vi "Handle Value Change.vi"(5 "VolatusAPI":refnum<class "VolatusAPI.lvclass">, 7 "CtlRef":refnum<vi>, 8 "error in (no error)":errorcluster, 9 "NewVal":variant, 10 "OldVal":variant, 11 "Sequencing Control in":refnum<class "Sequencing Control.lvclass">) -> (0 "error out":errorcluster, 3 "Sequencing Control out":refnum<class "Sequencing Control.lvclass">)   [LabVIEW 2020, in "VolatusSeqGUI.lvlib" / "Sequencing Control.lvclass"]
uses:
  Sequencing Control.lvclass
  Volatus/VolatusAPI/VolatusAPI.lvclass
  Action.ctl
  Action Data.ctl
  Sequencing Control.lvclass/Sequencing Control.ctl
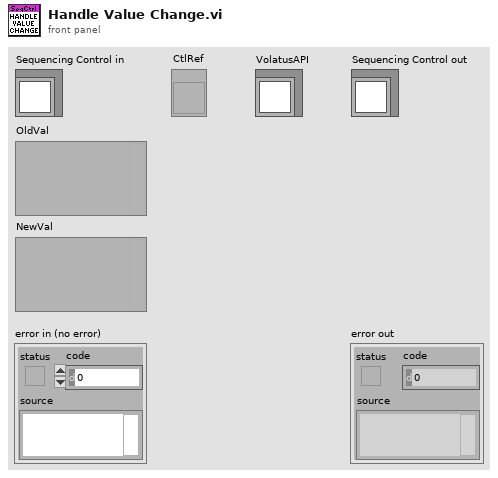
[diagram p1: front panel]
types:
  T1 = cluster{"Sequences":cluster{"Name Color":u32, "Name":string, "Btn 1 Color":u32, "Btn 1 Text":string, "Btn 2 Color":u32, "Btn 2 Text":string, "Status Color":u32, "Status":string, "State Time":string, "Started":string, "Seq Time":string, "Btn 1":bool, "Btn 2":bool, "Btn Name":bool}[], "Unload All":bool, "Abort All":bool, "Loaded, Good CRC":u32, "Sequence Error":u32, "Loaded, CRC Mismatch":u32, "Running, Good CRC":u32, "Unloaded":u32, "Running, CRC Mismatch":u32}
  T2 = cluster{"Sequences":cluster{"Name Color":bool, "Name":bool, "Btn 1 Color":bool, "Btn 1 Text":bool, "Btn 2 Color":bool, "Btn 2 Text":bool, "Status Color":bool, "Status":bool, "State Time":bool, "Started":bool, "Seq Time":bool, "Btn 1":bool, "Btn 2":bool, "Btn Name":bool}[], "Unload All":bool, "Abort All":bool, "Loaded, Good CRC":bool, "Sequence Error":bool, "Loaded, CRC Mismatch":bool, "Running, Good CRC":bool, "Unloaded":bool, "Running, CRC Mismatch":bool}
  T3 = cluster{"Name Color":u32, "Name":string, "Btn 1 Color":u32, "Btn 1 Text":string, "Btn 2 Color":u32, "Btn 2 Text":string, "Status Color":u32, "Status":string, "State Time":string, "Started":string, "Seq Time":string, "Btn 1":bool, "Btn 2":bool, "Btn Name":bool}[]
  T4 = cluster{"Name Color":bool, "Name":bool, "Btn 1 Color":bool, "Btn 1 Text":bool, "Btn 2 Color":bool, "Btn 2 Text":bool, "Status Color":bool, "Status":bool, "State Time":bool, "Started":bool, "Seq Time":bool, "Btn 1":bool, "Btn 2":bool, "Btn Name":bool}[]
  T5 = typedef "VolatusSeqGUI.lvlib/Sequencing Control.lvclass/Action.ctl" = enum16{"Details", "Load", "Unload", "Run", "Abort", "Unload All", "Abort All"}
  T6 = typedef "VolatusSeqGUI.lvlib/Sequencing Control.lvclass/Action Data.ctl" = cluster{"Action":T5, "Sequence":string}
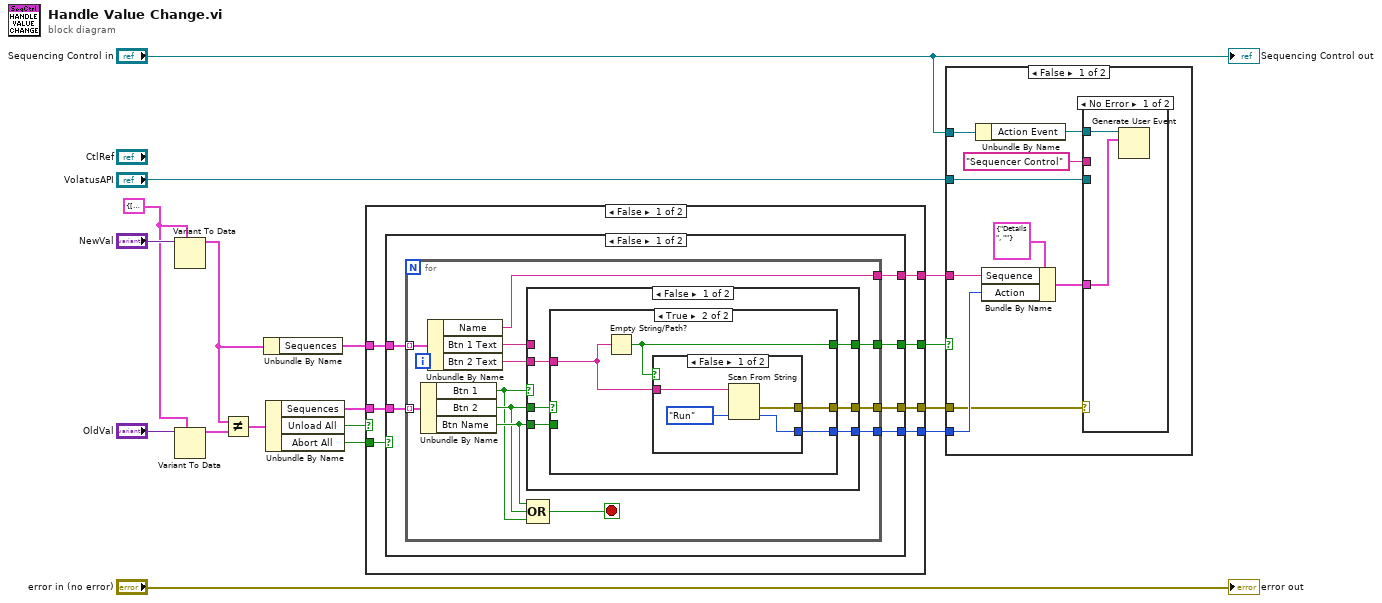
[diagram p0: block diagram]
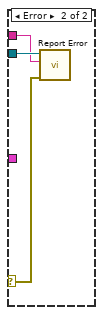
[diagram p2: hidden frame]
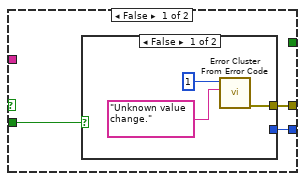
[diagram p4: hidden frame]
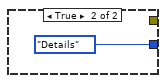
[diagram p5: hidden frame]
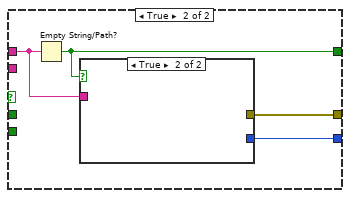
[diagram p7: hidden frame]
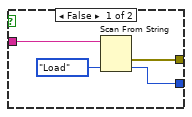
[diagram p8: hidden frame]
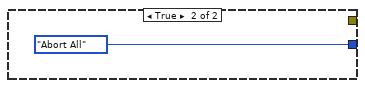
[diagram p9: hidden frame]
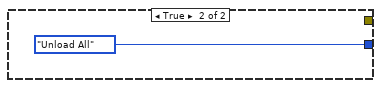
[diagram p10: hidden frame]
diagram:
  w14 = T1 {"Sequences"=[], "Unload All"=FALSE, "Abort All"=FALSE, "Loaded, Good CRC"=13816530, "Sequence Error"=16744319, "Loaded, CRC Mismatch"=16777142, "Running, Good CRC"=11730866, "Unloaded"=7171459, "Running, CRC Mismatch"=10530559} ("Sequencing")
  n1 = Variant To Data(type=w14, Variant="NewVal") -> (data=w8:T1)  [unwired: 1 in, 1 out]
  n2 = Variant To Data(type=w14, Variant="OldVal") -> (data=w13:T1)  [unwired: 1 in, 1 out]
  n3 = Not Equal?(x=w8, y=w13) -> (x != y?=w12:T2)
  n4 = Unbundle By Name(w8) -> ("Sequences"=w7:T3)
  n5 = Unbundle By Name(w12) -> ("Sequences"=w9:T4, "Unload All"=w11:bool, "Abort All"=w10:bool)
  n6 = case shown="False" w11 {
    tunnel: w10 -> [w24 _]
    tunnel: w9 -> [w22 _]
    tunnel: [w23 Action."Unload All" ("Action")] -> w5
    tunnel: w7 -> [w21 _]
    tunnel: [w20 _] -> w6
    tunnel: [w19 _] -> w3
    tunnel: [w18 _] -> w1
    frame False {
      n7 = case shown="False" w24 {
        tunnel: [w27 Action."Abort All" ("Action")] -> w23
        tunnel: w22 -> [w30 _]
        tunnel: w21 -> [w29 _]
        tunnel: [w28 _] -> w20
        tunnel: [w26 _] -> w19
        tunnel: [w25 _] -> w18
        frame False {
          n8 = for {
            tunnel: w30 -> [w42] mode=indexing
            tunnel: w29 -> [w41] mode=indexing
            tunnel: [w38] -> w28
            tunnel: [w37] -> w27
            tunnel: [w36] -> w26
            tunnel: [w31] -> w25
            stop <- w32 stop-if-true
            n9 = Unbundle By Name(w42) -> ("Btn 1"=w33:bool, "Btn 2"=w34:bool, "Btn Name"=w35:bool)
            n10 = Unbundle By Name(w41) -> ("Name"=w38:string, "Btn 1 Text"=w40:string, "Btn 2 Text"=w39:string)
            n11 = case shown="False" w33 {
              tunnel: w39 -> [w47 _]
              tunnel: [w44 w67] -> w37
              tunnel: [w46 w66] -> w36
              tunnel: w40 -> [_ w65]
              tunnel: w34 -> [w48 _]
              tunnel: w35 -> [w45 _]
              tunnel: [w43 w64] -> w31
              frame False {
                n12 = case shown="True" w48 {
                  tunnel: w47 -> [_ w57]
                  tunnel: [w49 w59] -> w46
                  tunnel: w45 -> [w51 _]
                  tunnel: [w50 w58] -> w44
                  tunnel: [_ w56] -> w43
                  frame False {
                    n13 = case shown="False" w51 {
                      tunnel: [_ Action."Details" ("Action")] -> w50
                      tunnel: [w54 _] -> w49
                      frame False {
                        n14 = call <vilib>:"Error Cluster From Error Code.vi"("error message (\"\")"="Unknown value change.", "error code (0)"=1) -> ("error out"=w54:errorcluster)  [unwired: 7 in]
                      }
                      frame True {
                      }
                    }
                  }
                  frame True {
                    n15 = Empty String/Path?(string/path=w57) -> (empty?=w56:bool)
                    n16 = case shown="False" w56 {
                      tunnel: [w63 _] -> w59
                      tunnel: [w61 _] -> w58
                      tunnel: w57 -> [w60 _]
                      frame False {
                        n17 = Scan From String(input string=w60, default 1=Action."Run" ("Action")) -> (error out=w63:errorcluster, output 1=w61:T5)  [unwired: 3 in, 2 out]
                      }
                      frame True {
                      }
                    }
                  }
                }
              }
              frame True {
                n18 = Empty String/Path?(string/path=w65) -> (empty?=w64:bool)
                n19 = case shown="True" w64 {
                  tunnel: [w70 _] -> w67
                  tunnel: [w69 _] -> w66
                  tunnel: w65 -> [w68 _]
                  frame False {
                    n20 = Scan From String(input string=w68, default 1=Action."Load" ("Action")) -> (error out=w69:errorcluster, output 1=w70:T5)  [unwired: 3 in, 2 out]
                  }
                  frame True {
                  }
                }
              }
            }
            n21 = Compound Arithmetic op=OR(w35, w34, w33) -> (w32:bool)
          }
        }
        frame True {
        }
      }
    }
    frame True {
    }
  }
  n22 = case shown="False" w1 {
    tunnel: w6 -> [w81 _]
    tunnel: w5 -> [w80 _]
    tunnel: "VolatusAPI" -> [w79 _]
    tunnel: w3 -> [w78 _]
    tunnel: "Sequencing Control in" -> [w76 _]
    frame False {
      n23 = Unbundle By Name(w76) -> ("Action Event"=w75:refnum<user-event>)
      n24 = Bundle By Name(cluster=T6 {"Action"=enum."Details", "Sequence"=""} ("Action Data"), "Sequence"=w81, "Action"=w80) -> (w77:T6)
      n25 = case shown="No Error" w78 {
        selector: w78 -> [_ w86]
        tunnel: w79 -> [_ w87]
        tunnel: w77 -> [w83 _]
        tunnel: w75 -> [w84 _]
        tunnel: "Sequencer Control" -> [_ w85]
        frame No Error {
          n26 = Generate User Event(user event=w84, event data cluster=w83) -> ()  [unwired: 2 in, 2 out]
        }
        frame Error {
          n27 = call "Report Error.vi"("error in (no error)"=w86, "Context"=w85, "VolatusAPI in"=w87) -> ()  [unwired: 7 in, 2 out]
        }
      }
    }
    frame True {
      # "Action skipped, no action available for button."
    }
  }
  "error out" <- "error in (no error)"
  "Sequencing Control out" <- "Sequencing Control in"
